vi "FindNodes.vi"(8 "error in (no error)":errorcluster, 9 "size":i32 caption="size (all)", 10 "Search":refnum<class "LLSearch.lvclass">, 11 "LinkedList in":refnum<class "LinkedList.lvclass">) -> (0 "error out":errorcluster, 1 "ignore":bool, 2 "LLNodes":refnum<data-value>[](array[refnum]), 3 "LinkedList out":refnum<class "LinkedList.lvclass">)   [LabVIEW 2009, in "LinkedList.lvclass"]
uses:
  LinkedList.lvclass
  LLNode/LLNode.lvclass
  LLSearch/LLSearch.lvclass
  Node/Node.lvclass
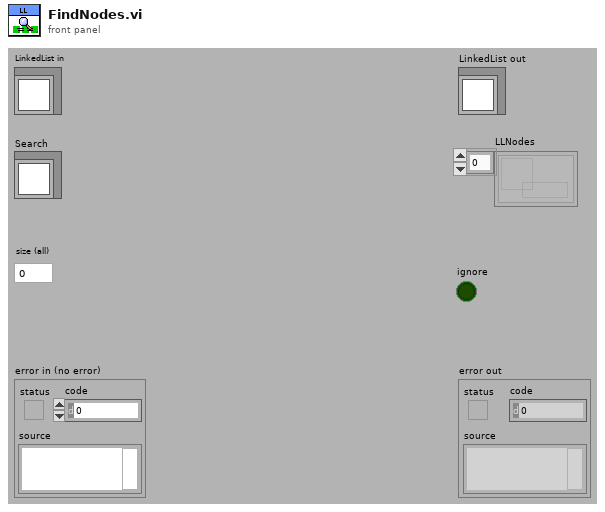
[diagram p1: front panel]
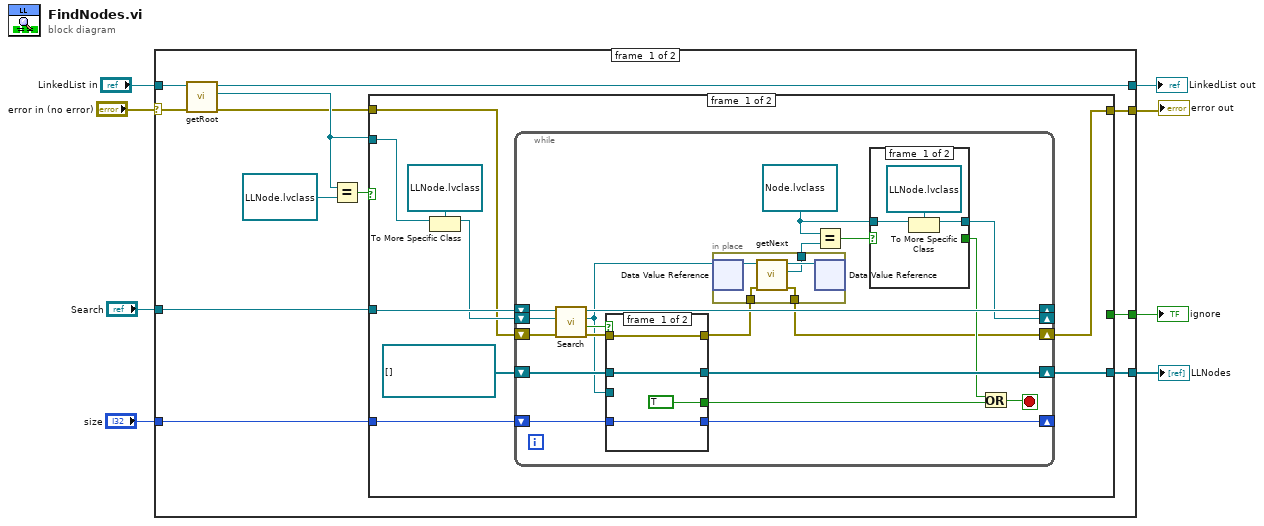
[diagram p0: block diagram]
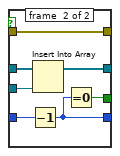
[diagram p3: hidden frame]
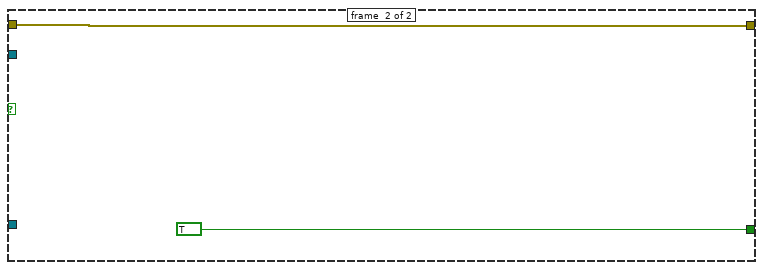
[diagram p4: hidden frame]
diagram:
  n1 = case shown="No Error" "error in (no error)" {
    selector: "error in (no error)" -> [w13 w72]
    tunnel: [w19 w73] -> w6
    tunnel: "LinkedList in" -> [w20 w73]
    tunnel: "Search" -> [w14 _]
    tunnel: "size" -> [w11 _]
    tunnel: [w15 _] -> w3
    tunnel: [w10 _] -> w2
    tunnel: [w9 w72] -> w1
    frame #0 {
      n2 = call "getRoot.vi"("error in (no error)"=w13, "LinkedList in"=w20) -> ("error out"=w12:errorcluster, "Root"=w16:refnum<data-value>, "LinkedList out"=w19:refnum<class "LinkedList.lvclass">)  [unwired: 7 in]
      n3 = Equal?(x=w16, y=refnum<data-value> refnum) -> (x = y?=w17:bool)
      n4 = case shown="False" w17 {
        tunnel: w16 -> [w29 _]
        tunnel: [_ TRUE] -> w15
        tunnel: w14 -> [w27 _]
        tunnel: w12 -> [w24 w70]
        tunnel: w11 -> [w25 _]
        tunnel: [w22 _] -> w10
        tunnel: [w21 w70] -> w9
        frame #0 {
          n5 = To More Specific Class(target class=refnum<data-value> refnum ("data value reference"), reference=w29) -> (specific class reference=w26:refnum<data-value>)  [unwired: 1 in, 1 out]
          n6 = while {
            shift-right: [w44] -> _
            shift-left: w27 -> [w49]
            shift-right: [w31] -> _
            shift-left: w26 -> [w48]
            shift-right: [w42] -> w22
            shift-left: refnum<data-value>[] [] -> [w43]
            shift-right: [w30] -> w21
            shift-left: w24 -> [w47]
            shift-right: [w40] -> _
            shift-left: w25 -> [w41]
            stop <- w35 stop-if-true
            w32 = refnum<data-value> refnum ("x")
            n7 = call "Search.vi"("error in (no error)"=w47, "LLNode in"=w48, "LLSearch in"=w49) -> ("error out"=w45:errorcluster, "found"=w46:bool, "LLNode out"=w39:refnum<data-value>, "LLSearch out"=w44:refnum<class "LLSearch.lvclass">)  [unwired: 5 in]
            n8 = case shown="True" w46 {
              tunnel: w45 -> [w60 w69]
              tunnel: [TRUE w67] -> w34
              tunnel: w43 -> [w61 w65]
              tunnel: [w61 w63] -> w42
              tunnel: [w60 w69] -> w38
              tunnel: w41 -> [w59 w68]
              tunnel: [w59 w66] -> w40
              tunnel: w39 -> [_ w64]
              frame #0 {
              }
              frame #1 {
                n9 = Decrement(x=w68) -> (x-1=w66:i32)
                n10 = Insert Into Array(array=w65, new element=w64) -> (w63:refnum<data-value>[])  [unwired: 1 in]
                n11 = Equal To 0?(x=w66) -> (x = 0?=w67:bool)
              }
            }
            n12 = in-place {
              in-place-border: w38 -> [w56]
              in-place-border: [w55] -> w30
              in-place-border: [w54] -> w37
              n13 = in-place-dvr #1(w39) -> (w58:refnum<class "LLNode.lvclass">)  [unwired: 1 out]
              n14 = call "getNext.vi"("error in (no error)"=w56, "LLNode in"=w58) -> ("error out"=w55:errorcluster, "next"=w54:refnum<data-value>, "LLNode out"=w57:refnum<class "LLNode.lvclass">)  [unwired: 7 in]
              n15 = in-place-dvr #1(w57) -> ()  [unwired: 2 out]
            }
            n16 = Equal?(x=w32, y=w37) -> (x = y?=w36:bool)
            n17 = case shown="False" w36 {
              selector: w36 -> [_ w53]
              tunnel: [_ w53] -> w33
              tunnel: w32 -> [w51 _]
              tunnel: [w50 _] -> w31
              frame #0 {
                n18 = To More Specific Class(target class=refnum<data-value> refnum ("data value reference"), reference=w51) -> (specific class reference=w50:refnum<data-value>)  [unwired: 1 in, 1 out]
              }
              frame #1 {
              }
            }
            n19 = Or(x=w33, y=w34) -> (x .or. y?=w35:bool)
          }
        }
        frame #1 {
        }
      }
    }
    frame #1 {
    }
  }
  "error out" <- w1
  "LinkedList out" <- w6
  "LLNodes" <- w2
  "ignore" <- w3
